vi "5207_Read_Channel1.vi"(3 "error in (no error)":errorcluster, 4 "Sensitivity (mV)":dbl, 5 "VISA resource name":refnum<visa-resource-name>) -> (0 "error out":errorcluster, 1 "Channel 1":dbl, 2 "VISA resource name out":refnum<visa-resource-name>)   [LabVIEW 2015]
panel:
  out "read buffer":string
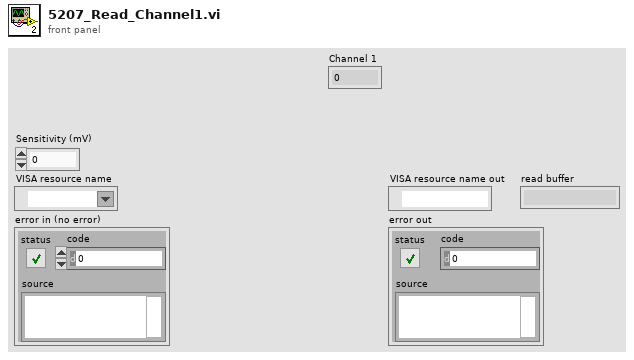
[diagram p1: front panel]
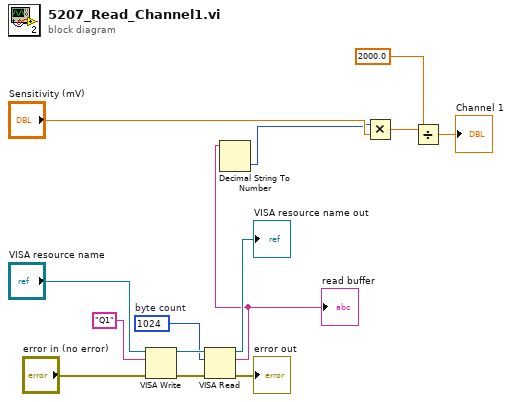
[diagram p0: block diagram]
diagram:
  w11 = u32 1024  # byte count
  n1 = VISA Write(VISA resource name="VISA resource name", write buffer="Q1" ("Write Buffer"), error in (no error)="error in (no error)") -> (VISA resource name out=w14:refnum<visa-resource-name>, error out=w13:errorcluster)  [unwired: 1 out]
  n2 = VISA Read(VISA resource name=w14, byte count=w11, error in (no error)=w13) -> (VISA resource name out=→"VISA resource name out":refnum<visa-resource-name>, read buffer=w5:string, error out=→"error out":errorcluster)  [unwired: 1 out]
  "read buffer" <- w5
  n3 = Decimal String To Number(string=w5) -> (number=w4:i32)  [unwired: 2 in, 1 out]
  n4 = Multiply(x=w4, y="Sensitivity (mV)") -> (x*y=w3:dbl)
  n5 = Divide(x=w3, y=2000.0) -> (x/y=→"Channel 1":dbl)
